vi "PH_PP_Common.get Trigger Tagname.vi"(1 "Trigger Tag":T2, 2 "PU":T1) -> (0 "Trigger Tagname":string)   [LabVIEW 2014, in "PH_PP_Common.lvlib"]
doc: "This VI concatenates a Tagname out of strict type def enum controls. It keeps also the information whether the Tag is existing (if not, N/A is given out as name)."
uses:
  PH_PP_Common.lvlib
  PH_PP_Common.Trigger Tags.ctl
  PH_PP_Common.PUs.ctl
  PH_Common/Names/PH_Names.Communication Type.ctl
  PH_Common/Names/PH_Names.Subsystems.ctl
  PH_PP_Common.Devices.ctl
  PH_Common/PH_Common.lvlib
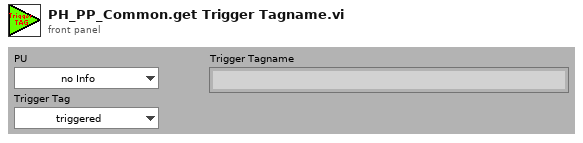
[diagram p1: front panel]
types:
  T1 = typedef "PH_PP_Common.lvlib/PH_PP_Common.PUs.ctl" = enum16{"no Info", "PA-19mm-1", "PA-19mm-2", "PA-45mm-PILC", "PA-45mm-MAIN", "MA-PU-1", "MA-PU-2", "MA-PU-3", "MA-PU-4", "MA-PU-5", "MA-PU-6", "MA-FR", "MA-PILC", "PA-45mm-DP"}
  T2 = typedef "PH_PP_Common.lvlib/PH_PP_Common.Trigger Tags.ctl" = enum16{"triggered", "fired", "Status", "Last Shot"}
  T3 = typedef "PH_Common.lvlib/PH_Names.Communication Type.ctl" = enum16{"no Info", "SE", "SA", "AE", "AA", "DE", "DA", "DIM"}
  T4 = typedef "PH_PP_Common.lvlib/PH_PP_Common.Devices.ctl" = enum16{"no Info", "Igni", "RR", "DumpRoss", "PSU", "Trigger", "HV-Meas", "Rods", "Chiller", "Conductivity", "Mercury"}
  T5 = typedef "PH_Common.lvlib/PH_Names.Subsystems.ctl" = enum16{"no Info", "fs-FE", "ns-FE", "PA", "MA", "MAS", "COS", "Exp-LB", "Exp-LL", "PP", "PILS"}
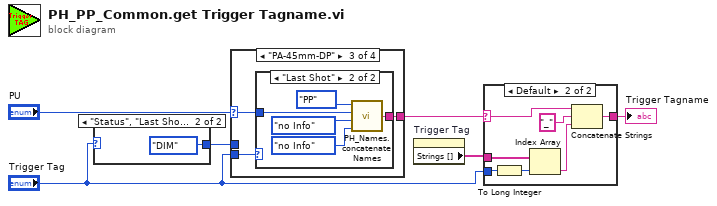
[diagram p0: block diagram]
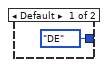
[diagram p2: hidden frame]
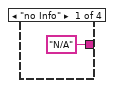
[diagram p3: hidden frame]
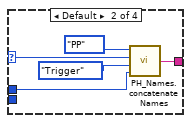
[diagram p4: hidden frame]
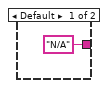
[diagram p5: hidden frame]
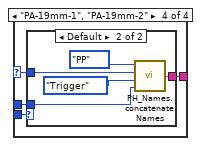
[diagram p6: hidden frame]
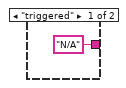
[diagram p7: hidden frame]
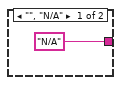
[diagram p8: hidden frame]
diagram:
  n1 = case shown="\"Status\", \"Last Shot\"" "Trigger Tag" {
    tunnel: [PH_Names.Communication_Type."DE" ("Communication Type (no info)") PH_Names.Communication_Type."DIM" ("Communication Type (no info)")] -> w2
    frame Default {
    }
    frame "Status", "Last Shot" {
    }
  }
  n2 = case shown="\"PA-45mm-DP\"" "PU" {
    selector: "PU" -> [_ w12 w16 w26]
    tunnel: ["N/A" ("Subsystem_PU_Devices_Comm Type") w14 w17 w27] -> w5
    tunnel: "Trigger Tag" -> [_ _ w15 w24]
    tunnel: w2 -> [_ w10 _ w25]
    frame "no Info" {
    }
    frame Default {
      n3 = call "PH_Names.concatenate Names.vi"("Communication Type (no info)"=w10, "Devices (no info)"=PH_PP_Common.Devices."Trigger", "PU (no info)"=w12, "Subsystem"=PH_Names.Subsystems."PP") -> ("Subsystem_PU_Devices_Comm Type"=w14:string)
    }
    frame "PA-45mm-DP" {
      n4 = case shown="\"Last Shot\"" w15 {
        tunnel: ["N/A" ("Subsystem_PU_Devices_Comm Type") w23] -> w17
        tunnel: w16 -> [_ w21]
        frame Default {
        }
        frame "Last Shot" {
          n5 = call "PH_Names.concatenate Names.vi"("Communication Type (no info)"=PH_Names.Communication_Type."no Info", "Devices (no info)"=PH_PP_Common.Devices."no Info", "PU (no info)"=w21, "Subsystem"=PH_Names.Subsystems."PP") -> ("Subsystem_PU_Devices_Comm Type"=w23:string)
        }
      }
    }
    frame "PA-19mm-1", "PA-19mm-2" {
      n6 = case shown="Default" w24 {
        tunnel: ["N/A" ("Subsystem_PU_Devices_Comm Type") w33] -> w27
        tunnel: w26 -> [_ w31]
        tunnel: w25 -> [_ w29]
        frame "triggered" {
        }
        frame Default {
          n7 = call "PH_Names.concatenate Names.vi"("Communication Type (no info)"=w29, "Devices (no info)"=PH_PP_Common.Devices."Trigger", "PU (no info)"=w31, "Subsystem"=PH_Names.Subsystems."PP") -> ("Subsystem_PU_Devices_Comm Type"=w33:string)
        }
      }
    }
  }
  n8 = property on="Trigger Tag" class="Enum (strict)"() -> ("Strings []"=w4:string[])  [unwired: 2 in, 2 out]
  n9 = case shown="Default" w5 {
    selector: w5 -> [_ w35]
    tunnel: ["N/A" w41] -> w6
    tunnel: w4 -> [_ w40]
    tunnel: "Trigger Tag" -> [_ w36]
    frame "", "N/A" {
    }
    frame Default {
      n10 = To Long Integer(number=w36) -> (32bit integer=w39:i32)
      n11 = Index Array(array=w40, index=w39) -> (element=w38:string)
      n12 = Concatenate Strings(w35, "_" ("string"), w38) -> (w41:string)
    }
  }
  "Trigger Tagname" <- w6
